vi "Connection Create.vi"(8 "error in (no error)":errorcluster, 11 "Ip : port":string) -> (0 "error out":errorcluster, 3 "Connection DVR out":refnum<data-value>)   [LabVIEW 2012, in "MDSplus.lvlib"]
uses:
  <vilib>/MDSplus/Library/MDSplus.lvlib
  <vilib>/MDSplus/Classes/Connection_Class/Connection.lvclass
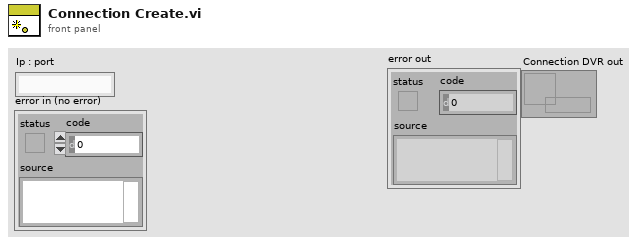
[diagram p1: front panel]
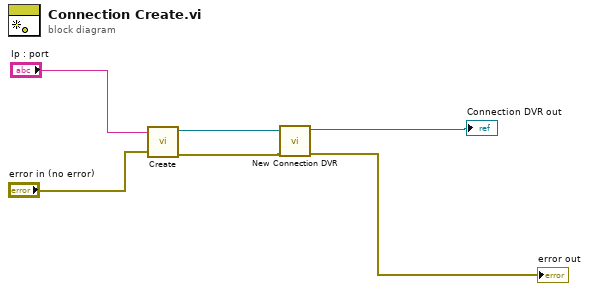
[diagram p0: block diagram]
diagram:
  n1 = call <vilib>:"Create.vi"("error in (no error)"="error in (no error)", "IP Address and Port"="Ip : port") -> ("error out"=w4:errorcluster, "Connection out"=w3:refnum<class "Connection.lvclass">)  [unwired: 8 in]
  n2 = call <vilib>:"New Connection DVR.vi"("error in (no error)"=w4, "Connection in"=w3) -> ("error out"=→"error out":errorcluster, "Connection DVR out"=→"Connection DVR out":refnum<data-value>)  [unwired: 8 in]
